vi "W3Q2.vi"() -> ()   [LabVIEW 2023]
panel:
  in  "Enum":T1(ring)
  out "result":dbl
  out "String":string
  in  "b":dbl
  in  "a":dbl
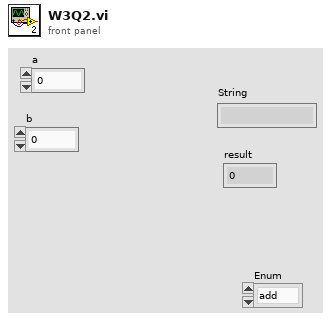
[diagram p1: front panel]
types:
  T1 = enum16{"add", "sub", "mul", "div", "sqr", "sqrt"}
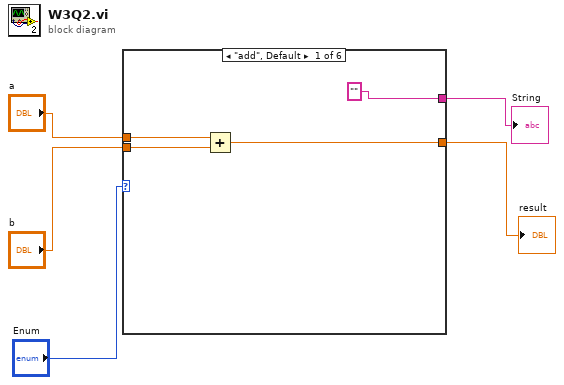
[diagram p0: block diagram]
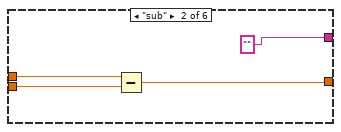
[diagram p2: hidden frame]
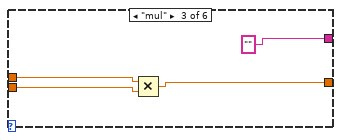
[diagram p3: hidden frame]
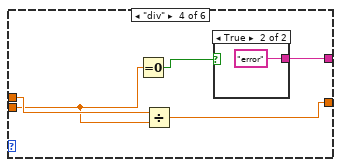
[diagram p4: hidden frame]
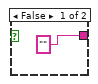
[diagram p5: hidden frame]
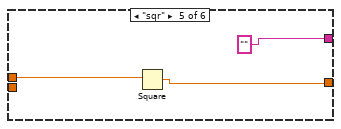
[diagram p6: hidden frame]
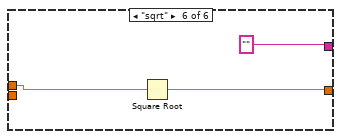
[diagram p7: hidden frame]
diagram:
  n1 = case shown="\"add\", Default" "Enum" {
    tunnel: "a" -> [w9 w13 w17 w22 w27 w30]
    tunnel: "b" -> [w8 w12 w16 w19 _ _]
    tunnel: [w7 w11 w15 w21 w26 w29] -> w2
    tunnel: ["" "" "" w20 "" ""] -> w1
    frame "add", Default {
      n2 = Add(x=w9, y=w8) -> (x+y=w7:dbl)
    }
    frame "sub" {
      n3 = Subtract(x=w13, y=w12) -> (x-y=w11:dbl)
    }
    frame "mul" {
      n4 = Multiply(x=w17, y=w16) -> (x*y=w15:dbl)
    }
    frame "div" {
      n5 = Equal To 0?(x=w19) -> (x = 0?=w18:bool)
      n6 = Divide(x=w22, y=w19) -> (x/y=w21:dbl)
      n7 = case shown="True" w18 {
        tunnel: ["" "error"] -> w20
        frame False {
        }
        frame True {
        }
      }
    }
    frame "sqr" {
      n8 = Square(x=w27) -> (x^2=w26:dbl)
    }
    frame "sqrt" {
      n9 = Square Root(x=w30) -> (sqrt(x)=w29:dbl)
    }
  }
  "String" <- w1
  "result" <- w2
